vi "Tach Edge Detection (No State).vi"(4 "state in":T1, 5 "reset? (True)":bool=TRUE, 6 "dt":dbl=11025.0, 8 "slope (Rising)":u16(ring) items=["Rising", "Falling"], 9 "pulse width (2)":i32=2, 10 "threshold (0.0)":dbl format="%.2f", 11 "x[n]":dbl[](array[numeric]) format="%.2f") -> (0 "state out":T1, 3 "pulse positions [s]":dbl[](array[numeric]) format="%.2f")   [LabVIEW 2017, in "VibrationAnalysisFunctions.lvlib"]
doc: "Detects the edges in the tachometer pulses contained in <B>x[n]</B> that cross <B>threshold</B>. Perform edge detection to determine the tachometer pulse position. The VI recognizes the points where the signal crosses <B>threshold</B> and <B>x[n]</B> as edges. The VI returns the locations of the detected edges in <B>pulse positions [s]</B>."
uses:
  <vilib>/addons/InsightCM/Utilities/Analysis/Vibration/VibrationAnalysisFunctions.lvlib
  <vilib>/Analysis/8numeric.llb/Threshold Detector.vi
  <vilib>/addons/Sound and Vibration/Order Analysis/Tach Process/SoundVib_TachProcess.lvlib
panel:
  # "Edge Detection (1 Tach)"
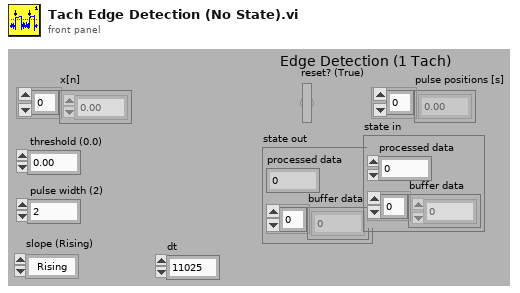
[diagram p1: front panel]
types:
  T1 = cluster{"processed data":dbl, "buffer data":dbl[]}
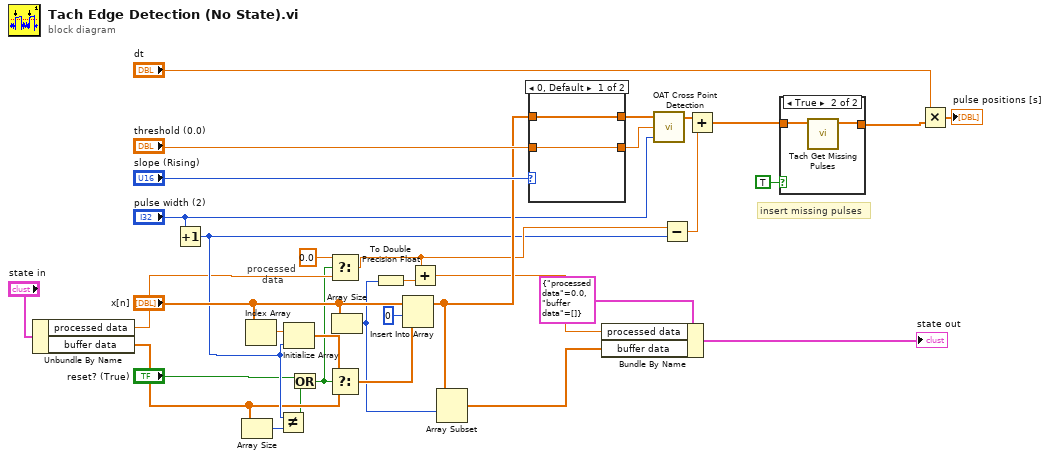
[diagram p0: block diagram]
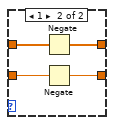
[diagram p3: hidden frame]
diagram:
  # "insert missing pulses"
  # "processed\n     data"
  n1 = Unbundle By Name("state in") -> ("processed data"=w16:dbl, "buffer data"=w15:dbl[])
  n2 = Increment(x="pulse width (2)") -> (x+1=w23:i32)
  n3 = Array Size(array=w15) -> (size(s)=w13:i32)
  n4 = Index Array(array="x[n]") -> (element=w14:dbl)  [unwired: 1 in]
  n5 = Not Equal?(x=w23, y=w13) -> (x != y?=w12:bool)
  n6 = Initialize Array(w14, w23) -> (w9:dbl[])
  n7 = Or(x="reset? (True)", y=w12) -> (x .or. y?=w8:bool)
  n8 = Select(t=0.0, s=w8, f=w16) -> (s? t:f=w26:dbl)
  n9 = Select(t=w9, s=w8, f=w15) -> (s? t:f=w11:dbl[])
  n10 = Array Size(array="x[n]") -> (size(s)=w6:i32)
  n11 = To Double Precision Float(number=w6) -> (double precision float=w5:dbl)
  n12 = Insert Into Array(array="x[n]", index=0 ("Index"), new element=w11) -> (w28:dbl[])
  n13 = Add(x=w26, y=w5) -> (x+y=w21:dbl)
  n14 = Array Subset(array=w28, index=w6) -> (w20:dbl[])  [unwired: 1 in]
  n15 = case shown="0, Default" "slope (Rising)" {
    tunnel: "threshold (0.0)" -> [w35 w38]
    tunnel: w28 -> [w36 w40]
    tunnel: [w36 w39] -> w31
    tunnel: [w35 w37] -> w33
    frame 0, Default {
    }
    frame 1 {
      n16 = Negate(x=w40) -> (-x=w39:dbl[])
      n17 = Negate(x=w38) -> (-x=w37:dbl)
    }
  }
  n18 = Bundle By Name(cluster=T1 {"processed data"=0.0, "buffer data"=[]}, "processed data"=w21, "buffer data"=w20) -> (→"state out":T1)
  n19 = call <vilib>:"OAT Cross Point Detection.vi"("pulse width (2)"="pulse width (2)", "threshold (0)"=w33, "data in"=w31) -> ("edge position"=w27:dbl[])  [unwired: 1 in]
  n20 = Subtract(x=w26, y=w23) -> (x-y=w24:dbl)
  n21 = Add(x=w27, y=w24) -> (x+y=w3:dbl[])
  n22 = case shown="True" TRUE {
    tunnel: w3 -> [w41 w43]
    tunnel: [w41 w42] -> w2
    frame False {
    }
    frame True {
      n23 = call <vilib>:"Tach Get Missing Pulses.vi"("pulse positions"=w43) -> ("modified pulse positions"=w42:dbl[])  [unwired: 9 in, 1 out]
    }
  }
  n24 = Multiply(x="dt", y=w2) -> (x*y=→"pulse positions [s]":dbl[])
